vi "MCSGlobalVarsWrite.vi"(2 "nOfBins":u32, 3 "nOfBunches":i32, 4 "MCSstate":T1, 5 "errorCount":i8, 10 "writeOnlyMCSState":bool, 11 "writeOnlyErrorCount":bool) -> ()   [LabVIEW 2014]
uses:
  Controls/MCSstate.ctl
  <vilib>/rvi/Emulation/niFpgaSctlEmulationGetInTimedLoop.vi
  MCSGlobalVars.vi
  <vilib>/rvi/Emulation/niFpgaProcessEmulError.vi
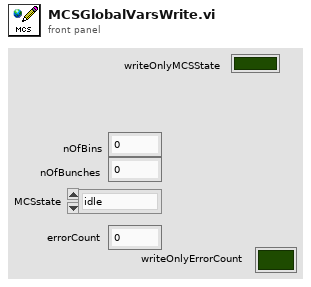
[diagram p1: front panel]
types:
  T1 = typedef "MCSstate.ctl" = enum16{"idle", "scanning", "done", "error"}
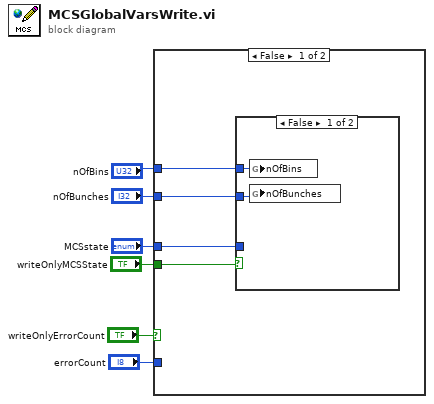
[diagram p0: block diagram]
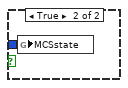
[diagram p2: hidden frame]
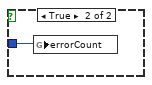
[diagram p3: hidden frame]
diagram:
  n1 = case shown="False" "writeOnlyErrorCount" {
    tunnel: "MCSstate" -> [w10 _]
    tunnel: "writeOnlyMCSState" -> [w9 _]
    tunnel: "nOfBins" -> [w8 _]
    tunnel: "nOfBunches" -> [w7 _]
    tunnel: "errorCount" -> [_ w14]
    frame False {
      n2 = case shown="False" w9 {
        tunnel: w10 -> [_ w13]
        tunnel: w8 -> [w12 _]
        tunnel: w7 -> [w11 _]
        frame False {
          n3 = global write "MCSGlobalVars.vi" "nOfBins"(w12) -> ()
          n4 = global write "MCSGlobalVars.vi" "nOfBunches"(w11) -> ()
        }
        frame True {
          n5 = global write "MCSGlobalVars.vi" "MCSstate"(w13) -> ()
        }
      }
    }
    frame True {
      n6 = global write "MCSGlobalVars.vi" "errorCount"(w14) -> ()
    }
  }
